vi "Drive_Vi.vi"(8 "Middle Thumb":bool, 9 "Z":dbl format="%#_13g", 10 "Y":dbl format="%#_13g", 11 "X":dbl format="%#_13g") -> ()   [LabVIEW 2020]
uses:
  <vilib>/Rock Robotics/WPI/ThirdParty/Phoenix-LabVIEW/Motor Controller/Controls/CTRE_Phoenix_MotorControl_ControlMode.ctl
  <vilib>/Rock Robotics/WPI/ThirdParty/Phoenix-LabVIEW/CANCoder/Get/CTRE_Phoenix_CANcoder_GetSensorData.vi
  <vilib>/Rock Robotics/WPI/ThirdParty/Phoenix-LabVIEW/Pigeon IMU/CTRE_PigeonIMU_GetYPR.vi
panel:
  in  "FR PID gains":T1={"proportional gain (Kc)"=0.01, "integral time (Ti, min)"=0.0, "derivative time (Td, min)"=0.0} {"derivative time (Td, min)" format="%.3f"; "integral time (Ti, min)" format="%.3f"; "proportional gain (Kc)" format="%.6f"}
  in  "FL PID gains":T1={"proportional gain (Kc)"=0.01, "integral time (Ti, min)"=0.0, "derivative time (Td, min)"=0.0} {"derivative time (Td, min)" format="%.3f"; "integral time (Ti, min)" format="%.3f"; "proportional gain (Kc)" format="%.6f"}
  in  "BR PID gains":T1={"proportional gain (Kc)"=0.01, "integral time (Ti, min)"=0.0, "derivative time (Td, min)"=0.0} {"derivative time (Td, min)" format="%.3f"; "integral time (Ti, min)" format="%.3f"; "proportional gain (Kc)" format="%.6f"}
  in  "BL PID gains":T1={"proportional gain (Kc)"=0.01, "integral time (Ti, min)"=0.0, "derivative time (Td, min)"=0.0} {"derivative time (Td, min)" format="%.3f"; "integral time (Ti, min)" format="%.3f"; "proportional gain (Kc)" format="%.6f"}
  out "BBC":dbl
  out "BFC":dbl
  out "OBC":dbl
  out "OFC":dbl
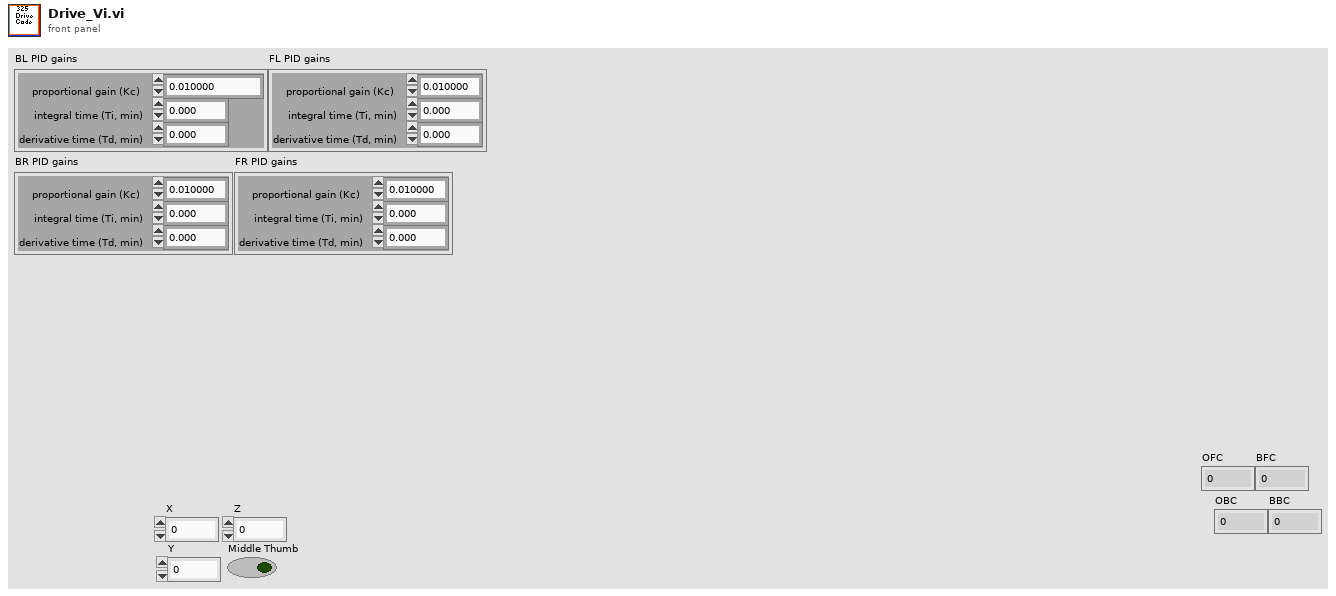
[diagram p1: front panel]
types:
  T1 = cluster{"proportional gain (Kc)":dbl, "integral time (Ti, min)":dbl, "derivative time (Td, min)":dbl}
  T2 = typedef "CTRE_Phoenix_MotorControl_ControlMode.ctl" = u16
  T3 = typedef "CTRE_PigeonIMU_DeviceRef.ctl" = cluster{"DeviceStatus":errorcluster, "Device Number":u8, "Type":T4, "Device ID":u32, "Handle":u64, "UsageFrame":u32, "Library Path":path}
  T4 = typedef "CTRE_PigeonIMU_ConnectionType.ctl" = u32
  T5 = typedef "CTRE_Phoenix_CANcoder_DeviceRef.ctl" = cluster{"DeviceStatus":errorcluster, "Device Number":u8, "Handle":u64, "UsageFrame":u32, "Library Path":path}
  T6 = typedef "WPI_MotorControlDeviceRef.ctl" = cluster{"DeviceStatus":errorcluster, "Type":T7, "PWM":cluster{"PWM Channel":T8, "DeadBand":T9}, "CAN":cluster{"Device Number":u8, "SetOutput VI Ref":variant, "GetOutput VI Ref":variant, "Enable VI Ref":variant, "Disable VI Ref":variant, "Data":variant}, "Invert":bool, "DIO PWM":cluster{"PWM \"Enable\" Channel":T8, "DIOChannel":T10, "PWM Rate":dbl}}
  T7 = typedef "WPI_MotorControlType.ctl" = enum16{"PWM", "CAN", "DIO PWM"}
  T8 = typedef "FPGA_DIOPWMChannel.ctl" = enum8{"PWM 0", "PWM 1", "PWM 2", "PWM 3", "PWM 4", "PWM 5", "PWM 6", "PWM 7", "PWM 8", "PWM 9", "PWM MXP 0", "PWM MXP 1", "PWM MXP 2", "PWM MXP 3", "PWM MXP 4", "PWM MXP 5", "PWM MXP 6", "PWM MXP 7", "PWM MXP 8", "PWM MXP 9", "Invalid"}
  T9 = typedef "WPI_PWMDeadband.ctl" = cluster{"Name":string, "maxPositivePwm":i32, "minPositivePwm":i32, "centerPwm":i32, "maxNegativePwm":i32, "minNegativePwm":i32, "angularRange":u16}
  T10 = typedef "FPGA_DIOChannel.ctl" = enum8{"DIO 0", "DIO 1", "DIO 2", "DIO 3", "DIO 4", "DIO 5", "DIO 6", "DIO 7", "DIO 8", "DIO 9", "DIO MXP 0", "DIO MXP 1", "DIO MXP 2", "DIO MXP 3", "DIO MXP 4", "DIO MXP 5", "DIO MXP 6", "DIO MXP 7", "DIO MXP 8", "DIO MXP 9", "DIO MXP 10", "DIO MXP 11", "DIO MXP 12", "DIO MXP 13", "DIO MXP 14", "DIO MXP 15", "SPI Port CS1", "SPI Port CS2", "SPI Port CS3", "SPI Port MISO", "SPI Port MOSI", "Invalid"}
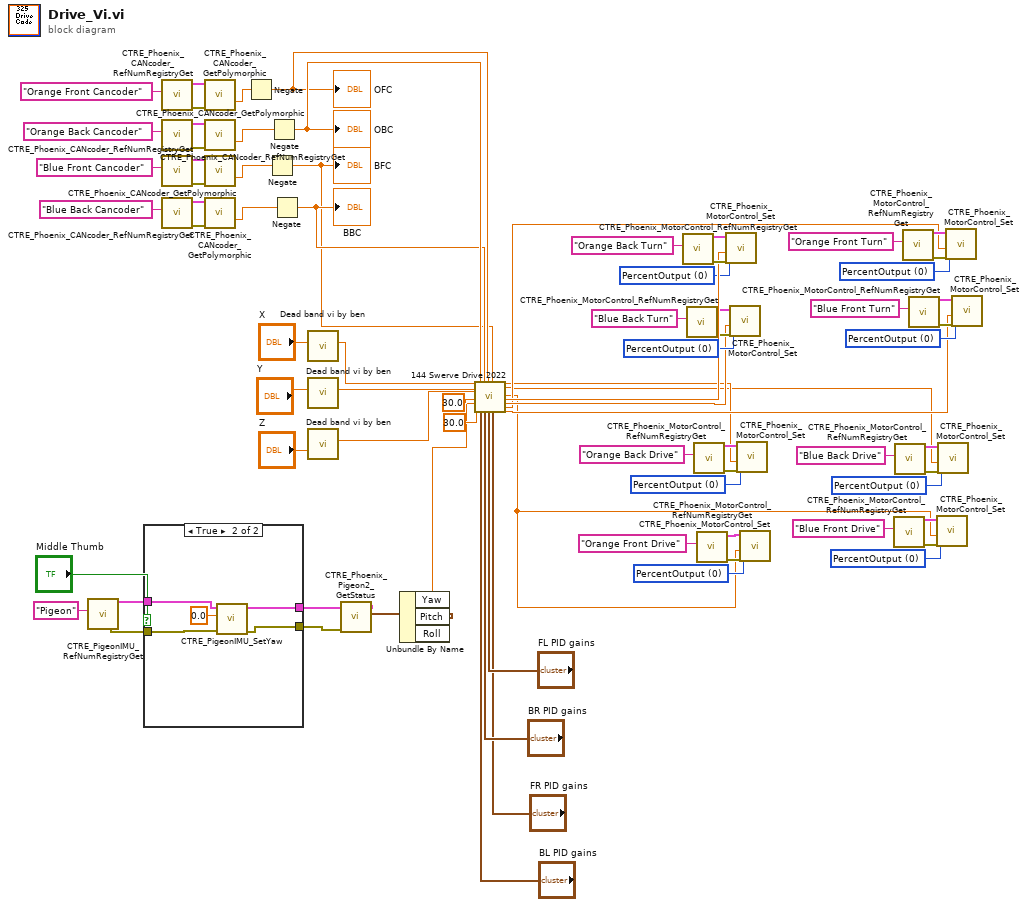
[diagram p0: block diagram]
diagram:
  w18 = T2 0 items=["PercentOutput"=0, "Position"=1, "Velocity"=2, "Current"=3, "Follower"=5, "MotionProfile"=6, "MotionMagic"=7, "MotionProfileArc"=10, "Disabled"=15] ("Control Mode")
  w22 = T2 0 items=["PercentOutput"=0, "Position"=1, "Velocity"=2, "Current"=3, "Follower"=5, "MotionProfile"=6, "MotionMagic"=7, "MotionProfileArc"=10, "Disabled"=15] ("Control Mode")
  w27 = T2 0 items=["PercentOutput"=0, "Position"=1, "Velocity"=2, "Current"=3, "Follower"=5, "MotionProfile"=6, "MotionMagic"=7, "MotionProfileArc"=10, "Disabled"=15] ("Control Mode")
  w32 = T2 0 items=["PercentOutput"=0, "Position"=1, "Velocity"=2, "Current"=3, "Follower"=5, "MotionProfile"=6, "MotionMagic"=7, "MotionProfileArc"=10, "Disabled"=15] ("Control Mode")
  w38 = T2 0 items=["PercentOutput"=0, "Position"=1, "Velocity"=2, "Current"=3, "Follower"=5, "MotionProfile"=6, "MotionMagic"=7, "MotionProfileArc"=10, "Disabled"=15] ("Control Mode")
  w43 = T2 0 items=["PercentOutput"=0, "Position"=1, "Velocity"=2, "Current"=3, "Follower"=5, "MotionProfile"=6, "MotionMagic"=7, "MotionProfileArc"=10, "Disabled"=15] ("Control Mode")
  w48 = T2 0 items=["PercentOutput"=0, "Position"=1, "Velocity"=2, "Current"=3, "Follower"=5, "MotionProfile"=6, "MotionMagic"=7, "MotionProfileArc"=10, "Disabled"=15] ("Control Mode")
  w56 = T2 0 items=["PercentOutput"=0, "Position"=1, "Velocity"=2, "Current"=3, "Follower"=5, "MotionProfile"=6, "MotionMagic"=7, "MotionProfileArc"=10, "Disabled"=15] ("Control Mode")
  n1 = call <vilib>:"CTRE_PigeonIMU_RefNumRegistryGet.vi"("refnum name"="Pigeon") -> ("error out"=w14:errorcluster, "PigeonIMUDevRef"=w15:T3)  [unwired: 9 in]
  n2 = case shown="True" "Middle Thumb" {
    tunnel: w15 -> [w81 w85]
    tunnel: w14 -> [w80 w84]
    tunnel: [w80 w83] -> w13
    tunnel: [w81 w82] -> w12
    frame False {
    }
    frame True {
      n3 = call <vilib>:"CTRE_PigeonIMU_SetYaw.vi"("error in (no error)"=w84, "Value"=0.0, "PigeonIMUDevRef"=w85) -> ("error out"=w83:errorcluster, "PigeonIMUDevRef"=w82:T3)  [unwired: 7 in]
    }
  }
  n4 = call <vilib>:"CTRE_Phoenix_CANcoder_RefNumRegistryGet.vi"("refnum name"="Orange Front Cancoder") -> ("error out"=w75:errorcluster, "CTRE_CANcoder_DeviceRef"=w76:T5)  [unwired: 9 in]
  n5 = call <vilib>:"CTRE_Phoenix_CANcoder_RefNumRegistryGet.vi"("refnum name"="Orange Back Cancoder") -> ("error out"=w73:errorcluster, "CTRE_CANcoder_DeviceRef"=w74:T5)  [unwired: 9 in]
  n6 = call <vilib>:"CTRE_Phoenix_CANcoder_RefNumRegistryGet.vi"("refnum name"="Blue Front Cancoder") -> ("error out"=w69:errorcluster, "CTRE_CANcoder_DeviceRef"=w70:T5)  [unwired: 9 in]
  n7 = call <vilib>:"CTRE_Phoenix_CANcoder_RefNumRegistryGet.vi"("refnum name"="Blue Back Cancoder") -> ("error out"=w71:errorcluster, "CTRE_CANcoder_DeviceRef"=w72:T5)  [unwired: 9 in]
  n8 = call-poly <vilib>:"CTRE_Phoenix_CANcoder_GetPolymorphic.vi"("CTRE_CANcoder_DeviceRef"=w76, "error in"=w75) -> ("Absolute Position"=w61:dbl)  [unwired: 9 in, 4 out]
  n9 = call-poly <vilib>:"CTRE_Phoenix_CANcoder_GetPolymorphic.vi"("CTRE_CANcoder_DeviceRef"=w74, "error in"=w73) -> ("Absolute Position"=w62:dbl)  [unwired: 9 in, 4 out]
  n10 = call-poly <vilib>:"CTRE_Phoenix_CANcoder_GetPolymorphic.vi"("CTRE_CANcoder_DeviceRef"=w70, "error in"=w69) -> ("Absolute Position"=w63:dbl)  [unwired: 9 in, 4 out]
  n11 = call-poly <vilib>:"CTRE_Phoenix_CANcoder_GetPolymorphic.vi"("CTRE_CANcoder_DeviceRef"=w72, "error in"=w71) -> ("Absolute Position"=w64:dbl)  [unwired: 9 in, 4 out]
  n12 = Negate(x=w61) -> (-x=w42:dbl)
  "OFC" <- w42
  n13 = Negate(x=w63) -> (-x=w35:dbl)
  "BFC" <- w35
  n14 = Negate(x=w62) -> (-x=w53:dbl)
  "OBC" <- w53
  n15 = Negate(x=w64) -> (-x=w52:dbl)
  "BBC" <- w52
  n16 = call "Dead band vi by ben.vi"("Numeric"="X") -> ("Deadbanded Value"=w79:dbl)  [unwired: 10 in]
  n17 = call "Dead band vi by ben.vi"("Numeric"="Y") -> ("Deadbanded Value"=w78:dbl)  [unwired: 10 in]
  n18 = call "Dead band vi by ben.vi"("Numeric"="Z") -> ("Deadbanded Value"=w77:dbl)  [unwired: 10 in]
  n19 = call-poly <vilib>:"CTRE_Phoenix_Pigeon2_GetStatus.vi"("error in (no error)"=w13, "PigeonIMUDevRef"=w12) -> ("Yaw Pitch Roll"=w10:cluster{"Yaw":dbl, "Pitch":dbl, "Roll":dbl})  [unwired: 7 in, 2 out]
  n20 = Unbundle By Name(w10) -> ("Yaw"=w9:dbl)  [unwired: 2 out]
  n21 = call "144 Swerve Drive 2022.vi"("Joystick X"=w79, "Joystick Y"=w78, "Joystick Z"=w77, "Robot Length(in.)"=30.0, "Robot Width(in.)"=30.0, "Gyro"=w9, "BL_Steer_Encoder"=w53, "BL PID gains"="BL PID gains", "BR_Steer_Encoder"=w52, "BR PID gains"="BR PID gains", "FL_Steer_Encoder"=w42, "FL PID gains"="FL PID gains", "FR_Steer_Encoder"=w35, "FR PID gains"="FR PID gains") -> ("Throttle BL"=w30:dbl, "Throttle BR"=w25:dbl, "Throttle FR"=w16:dbl, "BL_STEER_MOTOR_OUTPUT"=w57:dbl, "BR_STEER_MOTOR_OUTPUT"=w47:dbl, "FL_STEER_MOTOR_OUTPUT"=w37:dbl, "FR_STEER_MOTOR_OUTPUT"=w36:dbl)  [unwired: 6 in, 1 out]
  n22 = call <vilib>:"CTRE_Phoenix_MotorControl_RefNumRegistryGet.vi"("refnum name"="Orange Back Turn") -> ("error out"=w59:errorcluster, "PhoenixMotorControlDevRef"=w60:T6)  [unwired: 9 in]
  n23 = call <vilib>:"CTRE_Phoenix_MotorControl_RefNumRegistryGet.vi"("refnum name"="Blue Back Turn") -> ("error out"=w50:errorcluster, "PhoenixMotorControlDevRef"=w51:T6)  [unwired: 9 in]
  n24 = call <vilib>:"CTRE_Phoenix_MotorControl_RefNumRegistryGet.vi"("refnum name"="Orange Back Drive") -> ("error out"=w34:errorcluster, "PhoenixMotorControlDevRef"=w31:T6)  [unwired: 9 in]
  n25 = call <vilib>:"CTRE_Phoenix_MotorControl_RefNumRegistryGet.vi"("refnum name"="Orange Front Drive") -> ("error out"=w20:errorcluster, "PhoenixMotorControlDevRef"=w17:T6)  [unwired: 9 in]
  n26 = call <vilib>:"CTRE_Phoenix_MotorControl_Set.vi"("error in (no error)"=w59, "Output"=w57, "Control Mode"=w56, "PhoenixMotorControlDevRef"=w60) -> ()  [unwired: 6 in, 2 out]
  n27 = call <vilib>:"CTRE_Phoenix_MotorControl_Set.vi"("error in (no error)"=w50, "Output"=w47, "Control Mode"=w48, "PhoenixMotorControlDevRef"=w51) -> ()  [unwired: 6 in, 2 out]
  n28 = call <vilib>:"CTRE_Phoenix_MotorControl_Set.vi"("error in (no error)"=w34, "Output"=w30, "Control Mode"=w32, "PhoenixMotorControlDevRef"=w31) -> ()  [unwired: 6 in, 2 out]
  n29 = call <vilib>:"CTRE_Phoenix_MotorControl_Set.vi"("error in (no error)"=w20, "Output"=w16, "Control Mode"=w18, "PhoenixMotorControlDevRef"=w17) -> ()  [unwired: 6 in, 2 out]
  n30 = call <vilib>:"CTRE_Phoenix_MotorControl_RefNumRegistryGet.vi"("refnum name"="Blue Front Drive") -> ("error out"=w24:errorcluster, "PhoenixMotorControlDevRef"=w21:T6)  [unwired: 9 in]
  n31 = call <vilib>:"CTRE_Phoenix_MotorControl_RefNumRegistryGet.vi"("refnum name"="Blue Back Drive") -> ("error out"=w29:errorcluster, "PhoenixMotorControlDevRef"=w26:T6)  [unwired: 9 in]
  n32 = call <vilib>:"CTRE_Phoenix_MotorControl_RefNumRegistryGet.vi"("refnum name"="Orange Front Turn") -> ("error out"=w45:errorcluster, "PhoenixMotorControlDevRef"=w46:T6)  [unwired: 9 in]
  n33 = call <vilib>:"CTRE_Phoenix_MotorControl_RefNumRegistryGet.vi"("refnum name"="Blue Front Turn") -> ("error out"=w40:errorcluster, "PhoenixMotorControlDevRef"=w41:T6)  [unwired: 9 in]
  n34 = call <vilib>:"CTRE_Phoenix_MotorControl_Set.vi"("error in (no error)"=w24, "Output"=w16, "Control Mode"=w22, "PhoenixMotorControlDevRef"=w21) -> ()  [unwired: 6 in, 2 out]
  n35 = call <vilib>:"CTRE_Phoenix_MotorControl_Set.vi"("error in (no error)"=w29, "Output"=w25, "Control Mode"=w27, "PhoenixMotorControlDevRef"=w26) -> ()  [unwired: 6 in, 2 out]
  n36 = call <vilib>:"CTRE_Phoenix_MotorControl_Set.vi"("error in (no error)"=w45, "Output"=w37, "Control Mode"=w43, "PhoenixMotorControlDevRef"=w46) -> ()  [unwired: 6 in, 2 out]
  n37 = call <vilib>:"CTRE_Phoenix_MotorControl_Set.vi"("error in (no error)"=w40, "Output"=w36, "Control Mode"=w38, "PhoenixMotorControlDevRef"=w41) -> ()  [unwired: 6 in, 2 out]
